vi "ActiveSGChannels.vi"(4 "SG_data":T1[](array[typedef])) -> (1 "ActiveChannels":i32)   [LabVIEW 2016]
uses:
  StrainGauge/SG_data.ctl
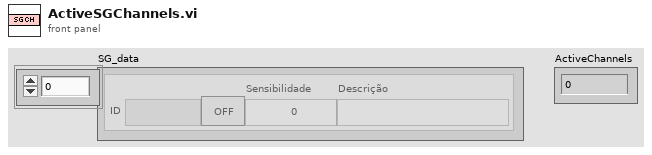
[diagram p1: front panel]
types:
  T1 = typedef "SG_data.ctl" = cluster{"ID":string, "Sensibilidade":dbl, "Descrição":string, "active":bool}
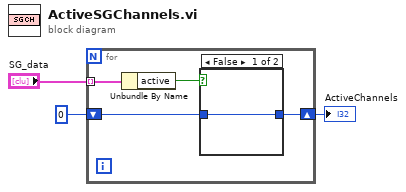
[diagram p0: block diagram]
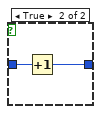
[diagram p2: hidden frame]
diagram:
  n1 = for {
    tunnel: "SG_data" -> [w7] mode=indexing
    shift-right: [w4] -> w3
    shift-left: 0 -> [w5]
    n2 = Unbundle By Name(w7) -> ("active"=w6:bool)
    n3 = case shown="False" w6 {
      tunnel: w5 -> [w8 w10]
      tunnel: [w8 w9] -> w4
      frame False {
      }
      frame True {
        n4 = Increment(x=w10) -> (x+1=w9:i32)
      }
    }
  }
  "ActiveChannels" <- w3
